vi "英维克空调告警存储.vi"   [LabVIEW 2016, in "环境动力监测库.lvlib" / "空调库.lvlib"]
uses:
  <vilib>/ptbypt/NI_PtbyPt.lvlib
types:
  T1 = cluster{"时间标识":timestamp, "设备":string, "日志信息":string}
  T2 = cluster{"高温告警":bool, "低温告警":bool, "高湿告警":bool, "低湿告警":bool, "盘管防冻":bool, "排气高温":bool, "盘管温感失效":bool, "室外温感失效":bool, "冷凝温感失效":bool, "内温感失效":bool, "排气温感失效":bool, "湿感失效":bool, "内风机故障":bool, "外风机故障":bool, "压缩机故障":bool, "电加热故障":bool, "应急风机故障":bool, "高压告警":bool, "低压告警":bool, "水浸告警":bool, "烟感告警":bool, "门禁告警":bool, "高压锁定":bool, "低压锁定":bool, "排气锁定":bool, "交流过压":bool, "交流欠压":bool, "交流掉压":bool, "缺相":bool, "频率异常":bool, "逆相":bool, "直流过压":bool, "直流欠压":bool}
  T3 = cluster{"漏水监测输出":cluster{"漏水监测告警":bool, "告警内容":string}, "门禁监测输出":cluster{"门禁监测告警":bool, "告警内容":string}, "门禁监测输出2":cluster{"门禁监测告警":bool, "告警内容":string}, "温湿度监测输出":cluster{"温湿度监测告警":bool, "告警内容":string}, "烟雾监测输出":cluster{"烟雾监测告警":bool, "告警内容":string}, "空调监测输出":cluster{"空调监测告警":bool, "告警内容":string}, "自动重合闸输出":cluster{"自动重合闸告警":bool, "告警内容":string}, "红外入侵输出":cluster{"红外入侵告警":bool, "告警内容":string}, "振动输出":cluster{"振动告警":bool, "告警内容":string}, "UPS输出":cluster{"UPS告警":bool, "告警内容":string}, "蓄电池输出":cluster{"蓄电池告警":bool, "告警内容":string}, "蓄电池输出2":cluster{"蓄电池告警":bool, "告警内容":string}, "GPS输出":cluster{"定位告警":bool, "告警内容":string}, "北斗输出":cluster{"定位告警":bool, "告警内容":string}, "气象输出":cluster{"气象告警":bool, "告警内容":string}}
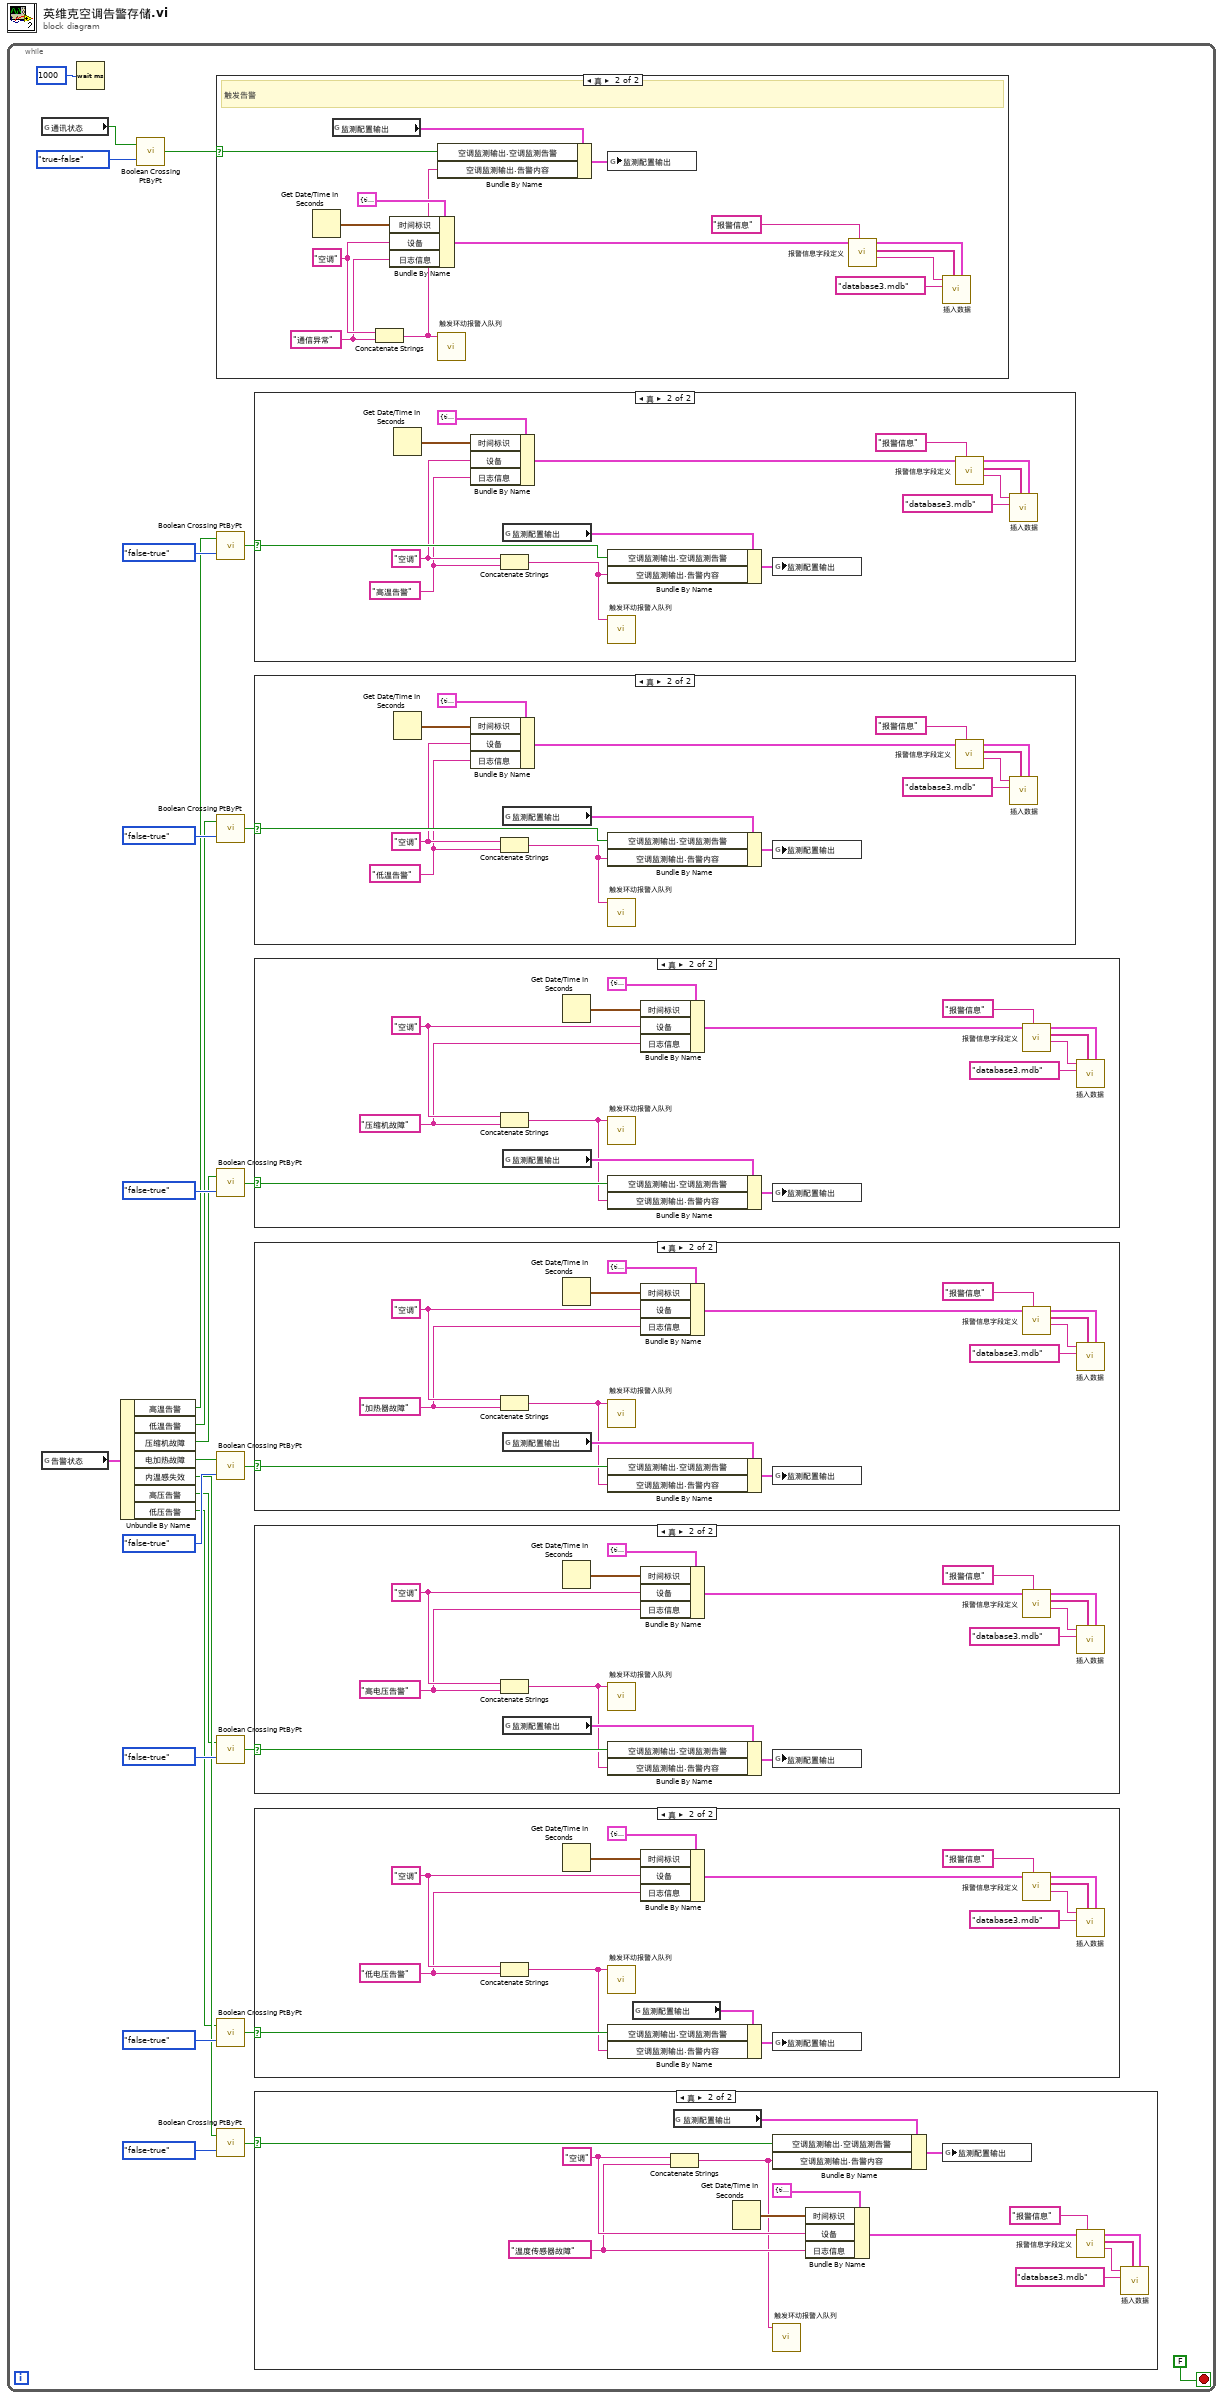
[diagram p0: block diagram]
diagram:
  n1 = while {
    stop <- FALSE stop-if-true
    n2 = global read "断电保存全局变量.vi" "通讯状态"() -> (w9:bool)
    n3 = global read "内部交互全局变量.vi" "告警状态"() -> (w8:T2)
    n4 = Wait (ms)(milliseconds to wait=u32 1000 ("等待时间（毫秒）")) -> ()  [unwired: 1 out]
    n5 = Unbundle By Name(w8) -> ("高温告警"=w6:bool, "低温告警"=w5:bool, "压缩机故障"=w7:bool, "电加热故障"=w4:bool, "内温感失效"=w3:bool, "高压告警"=w2:bool, "低压告警"=w1:bool)
    n6 = call <vilib>:"Boolean Crossing PtByPt.vi"("direction"=enum16{"either", "false-true", "true-false"}."true-false", "input"=w9) -> ("crossing"=w24:bool)  [unwired: 1 in]
    n7 = case shown="真" w24 {
      selector: w24 -> [_ w126]
      frame False {
      }
      frame True {
        w128 = "通信异常" ("日志信息")
        w129 = "空调" ("设备")
        # "触发告警"
        n8 = Get Date/Time In Seconds() -> (seconds since 1Jan1904=w139:timestamp)
        n9 = global read "断电保存全局变量.vi" "监测配置输出"() -> (w130:T3)
        n10 = Concatenate Strings(w129, w128) -> (w127:string)
        n11 = Bundle By Name(cluster=T1 {"时间标识"=timestamp(0 s since 1904-01-01), "设备"="", "日志信息"=""} ("data in"), "时间标识"=w139, "设备"=w129, "日志信息"=w128) -> (w138:T1)
        n12 = Bundle By Name(cluster=w130, "空调监测输出.空调监测告警"=w126, "空调监测输出.告警内容"=w127) -> (w131:T3)
        n13 = call "触发环动报警入队列.vi"("报警内容"=w127) -> ()  [unwired: 11 in]
        n14 = global write "断电保存全局变量.vi" "监测配置输出"(w131) -> ()
        n15 = call "报警信息字段定义.vi"("table输入"="报警信息", "data in"=w138) -> ("table输出"=w134:string, "columns"=w133:string[], "data out"=w132:T1)  [unwired: 7 in]
        n16 = call "插入数据.vi"("data"=w132, "columns"=w133, "database"="database3.mdb", "table"=w134) -> ()  [unwired: 7 in, 1 out]
      }
    }
    n17 = call <vilib>:"Boolean Crossing PtByPt.vi"("direction"=enum16{"either", "false-true", "true-false"}."false-true", "input"=w6) -> ("crossing"=w20:bool)  [unwired: 1 in]
    n18 = call <vilib>:"Boolean Crossing PtByPt.vi"("direction"=enum16{"either", "false-true", "true-false"}."false-true", "input"=w5) -> ("crossing"=w18:bool)  [unwired: 1 in]
    n19 = call <vilib>:"Boolean Crossing PtByPt.vi"("direction"=enum16{"either", "false-true", "true-false"}."false-true", "input"=w7) -> ("crossing"=w22:bool)  [unwired: 1 in]
    n20 = call <vilib>:"Boolean Crossing PtByPt.vi"("direction"=enum16{"either", "false-true", "true-false"}."false-true", "input"=w4) -> ("crossing"=w16:bool)  [unwired: 1 in]
    n21 = call <vilib>:"Boolean Crossing PtByPt.vi"("direction"=enum16{"either", "false-true", "true-false"}."false-true", "input"=w2) -> ("crossing"=w12:bool)  [unwired: 1 in]
    n22 = call <vilib>:"Boolean Crossing PtByPt.vi"("direction"=enum16{"either", "false-true", "true-false"}."false-true", "input"=w1) -> ("crossing"=w10:bool)  [unwired: 1 in]
    n23 = call <vilib>:"Boolean Crossing PtByPt.vi"("direction"=enum16{"either", "false-true", "true-false"}."false-true", "input"=w3) -> ("crossing"=w14:bool)  [unwired: 1 in]
    n24 = case shown="真" w20 {
      selector: w20 -> [_ w101]
      frame False {
      }
      frame True {
        w99 = "高温告警" ("日志信息")
        w100 = "空调" ("设备")
        n25 = Get Date/Time In Seconds() -> (seconds since 1Jan1904=w111:timestamp)
        n26 = Bundle By Name(cluster=T1 {"时间标识"=timestamp(0 s since 1904-01-01), "设备"="", "日志信息"=""} ("data in"), "时间标识"=w111, "设备"=w100, "日志信息"=w99) -> (w110:T1)
        n27 = Concatenate Strings(w100, w99) -> (w98:string)
        n28 = global read "断电保存全局变量.vi" "监测配置输出"() -> (w102:T3)
        n29 = Bundle By Name(cluster=w102, "空调监测输出.空调监测告警"=w101, "空调监测输出.告警内容"=w98) -> (w103:T3)
        n30 = call "触发环动报警入队列.vi"("报警内容"=w98) -> ()  [unwired: 11 in]
        n31 = global write "断电保存全局变量.vi" "监测配置输出"(w103) -> ()
        n32 = call "报警信息字段定义.vi"("table输入"="报警信息", "data in"=w110) -> ("table输出"=w106:string, "columns"=w105:string[], "data out"=w104:T1)  [unwired: 7 in]
        n33 = call "插入数据.vi"("data"=w104, "columns"=w105, "database"="database3.mdb", "table"=w106) -> ()  [unwired: 7 in, 1 out]
      }
    }
    n34 = case shown="真" w18 {
      selector: w18 -> [_ w87]
      frame False {
      }
      frame True {
        w85 = "低温告警" ("日志信息")
        w86 = "空调" ("设备")
        n35 = Get Date/Time In Seconds() -> (seconds since 1Jan1904=w97:timestamp)
        n36 = Bundle By Name(cluster=T1 {"时间标识"=timestamp(0 s since 1904-01-01), "设备"="", "日志信息"=""} ("data in"), "时间标识"=w97, "设备"=w86, "日志信息"=w85) -> (w96:T1)
        n37 = Concatenate Strings(w86, w85) -> (w84:string)
        n38 = global read "断电保存全局变量.vi" "监测配置输出"() -> (w88:T3)
        n39 = Bundle By Name(cluster=w88, "空调监测输出.空调监测告警"=w87, "空调监测输出.告警内容"=w84) -> (w89:T3)
        n40 = call "触发环动报警入队列.vi"("报警内容"=w84) -> ()  [unwired: 11 in]
        n41 = global write "断电保存全局变量.vi" "监测配置输出"(w89) -> ()
        n42 = call "报警信息字段定义.vi"("table输入"="报警信息", "data in"=w96) -> ("table输出"=w92:string, "columns"=w91:string[], "data out"=w90:T1)  [unwired: 7 in]
        n43 = call "插入数据.vi"("data"=w90, "columns"=w91, "database"="database3.mdb", "table"=w92) -> ()  [unwired: 7 in, 1 out]
      }
    }
    n44 = case shown="真" w22 {
      selector: w22 -> [_ w115]
      frame False {
      }
      frame True {
        w113 = "压缩机故障" ("日志信息")
        w114 = "空调" ("设备")
        n45 = Concatenate Strings(w114, w113) -> (w112:string)
        n46 = global read "断电保存全局变量.vi" "监测配置输出"() -> (w116:T3)
        n47 = Get Date/Time In Seconds() -> (seconds since 1Jan1904=w125:timestamp)
        n48 = call "触发环动报警入队列.vi"("报警内容"=w112) -> ()  [unwired: 11 in]
        n49 = Bundle By Name(cluster=w116, "空调监测输出.空调监测告警"=w115, "空调监测输出.告警内容"=w112) -> (w117:T3)
        n50 = Bundle By Name(cluster=T1 {"时间标识"=timestamp(0 s since 1904-01-01), "设备"="", "日志信息"=""} ("data in"), "时间标识"=w125, "设备"=w114, "日志信息"=w113) -> (w124:T1)
        n51 = global write "断电保存全局变量.vi" "监测配置输出"(w117) -> ()
        n52 = call "报警信息字段定义.vi"("table输入"="报警信息", "data in"=w124) -> ("table输出"=w120:string, "columns"=w119:string[], "data out"=w118:T1)  [unwired: 7 in]
        n53 = call "插入数据.vi"("data"=w118, "columns"=w119, "database"="database3.mdb", "table"=w120) -> ()  [unwired: 7 in, 1 out]
      }
    }
    n54 = case shown="真" w16 {
      selector: w16 -> [_ w73]
      frame False {
      }
      frame True {
        w71 = "加热器故障" ("日志信息")
        w72 = "空调" ("设备")
        n55 = Concatenate Strings(w72, w71) -> (w70:string)
        n56 = global read "断电保存全局变量.vi" "监测配置输出"() -> (w74:T3)
        n57 = Get Date/Time In Seconds() -> (seconds since 1Jan1904=w83:timestamp)
        n58 = call "触发环动报警入队列.vi"("报警内容"=w70) -> ()  [unwired: 11 in]
        n59 = Bundle By Name(cluster=w74, "空调监测输出.空调监测告警"=w73, "空调监测输出.告警内容"=w70) -> (w75:T3)
        n60 = Bundle By Name(cluster=T1 {"时间标识"=timestamp(0 s since 1904-01-01), "设备"="", "日志信息"=""} ("data in"), "时间标识"=w83, "设备"=w72, "日志信息"=w71) -> (w82:T1)
        n61 = global write "断电保存全局变量.vi" "监测配置输出"(w75) -> ()
        n62 = call "报警信息字段定义.vi"("table输入"="报警信息", "data in"=w82) -> ("table输出"=w78:string, "columns"=w77:string[], "data out"=w76:T1)  [unwired: 7 in]
        n63 = call "插入数据.vi"("data"=w76, "columns"=w77, "database"="database3.mdb", "table"=w78) -> ()  [unwired: 7 in, 1 out]
      }
    }
    n64 = case shown="真" w12 {
      selector: w12 -> [_ w45]
      frame False {
      }
      frame True {
        w43 = "高电压告警" ("日志信息")
        w44 = "空调" ("设备")
        n65 = Concatenate Strings(w44, w43) -> (w42:string)
        n66 = global read "断电保存全局变量.vi" "监测配置输出"() -> (w46:T3)
        n67 = Get Date/Time In Seconds() -> (seconds since 1Jan1904=w55:timestamp)
        n68 = call "触发环动报警入队列.vi"("报警内容"=w42) -> ()  [unwired: 11 in]
        n69 = Bundle By Name(cluster=w46, "空调监测输出.空调监测告警"=w45, "空调监测输出.告警内容"=w42) -> (w47:T3)
        n70 = Bundle By Name(cluster=T1 {"时间标识"=timestamp(0 s since 1904-01-01), "设备"="", "日志信息"=""} ("data in"), "时间标识"=w55, "设备"=w44, "日志信息"=w43) -> (w54:T1)
        n71 = global write "断电保存全局变量.vi" "监测配置输出"(w47) -> ()
        n72 = call "报警信息字段定义.vi"("table输入"="报警信息", "data in"=w54) -> ("table输出"=w50:string, "columns"=w49:string[], "data out"=w48:T1)  [unwired: 7 in]
        n73 = call "插入数据.vi"("data"=w48, "columns"=w49, "database"="database3.mdb", "table"=w50) -> ()  [unwired: 7 in, 1 out]
      }
    }
    n74 = case shown="真" w10 {
      selector: w10 -> [_ w31]
      frame False {
      }
      frame True {
        w29 = "低电压告警" ("日志信息")
        w30 = "空调" ("设备")
        n75 = Concatenate Strings(w30, w29) -> (w28:string)
        n76 = Get Date/Time In Seconds() -> (seconds since 1Jan1904=w41:timestamp)
        n77 = call "触发环动报警入队列.vi"("报警内容"=w28) -> ()  [unwired: 11 in]
        n78 = global read "断电保存全局变量.vi" "监测配置输出"() -> (w32:T3)
        n79 = Bundle By Name(cluster=w32, "空调监测输出.空调监测告警"=w31, "空调监测输出.告警内容"=w28) -> (w33:T3)
        n80 = Bundle By Name(cluster=T1 {"时间标识"=timestamp(0 s since 1904-01-01), "设备"="", "日志信息"=""} ("data in"), "时间标识"=w41, "设备"=w30, "日志信息"=w29) -> (w40:T1)
        n81 = global write "断电保存全局变量.vi" "监测配置输出"(w33) -> ()
        n82 = call "报警信息字段定义.vi"("table输入"="报警信息", "data in"=w40) -> ("table输出"=w36:string, "columns"=w35:string[], "data out"=w34:T1)  [unwired: 7 in]
        n83 = call "插入数据.vi"("data"=w34, "columns"=w35, "database"="database3.mdb", "table"=w36) -> ()  [unwired: 7 in, 1 out]
      }
    }
    n84 = case shown="真" w14 {
      selector: w14 -> [_ w59]
      frame False {
      }
      frame True {
        w57 = "温度传感器故障" ("日志信息")
        w58 = "空调" ("设备")
        n85 = Concatenate Strings(w58, w57) -> (w56:string)
        n86 = global read "断电保存全局变量.vi" "监测配置输出"() -> (w60:T3)
        n87 = Get Date/Time In Seconds() -> (seconds since 1Jan1904=w69:timestamp)
        n88 = Bundle By Name(cluster=w60, "空调监测输出.空调监测告警"=w59, "空调监测输出.告警内容"=w56) -> (w61:T3)
        n89 = call "触发环动报警入队列.vi"("报警内容"=w56) -> ()  [unwired: 11 in]
        n90 = Bundle By Name(cluster=T1 {"时间标识"=timestamp(0 s since 1904-01-01), "设备"="", "日志信息"=""} ("data in"), "时间标识"=w69, "设备"=w58, "日志信息"=w57) -> (w68:T1)
        n91 = global write "断电保存全局变量.vi" "监测配置输出"(w61) -> ()
        n92 = call "报警信息字段定义.vi"("table输入"="报警信息", "data in"=w68) -> ("table输出"=w64:string, "columns"=w63:string[], "data out"=w62:T1)  [unwired: 7 in]
        n93 = call "插入数据.vi"("data"=w62, "columns"=w63, "database"="database3.mdb", "table"=w64) -> ()  [unwired: 7 in, 1 out]
      }
    }
  }
